vi "Set File Path.vi"(8 "error in":errorcluster) -> (0 "error out":errorcluster, 3 "path":path)   [LabVIEW 2018]
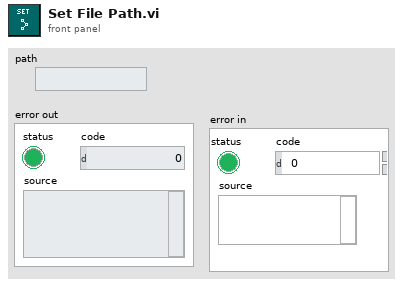
[diagram p1: front panel]
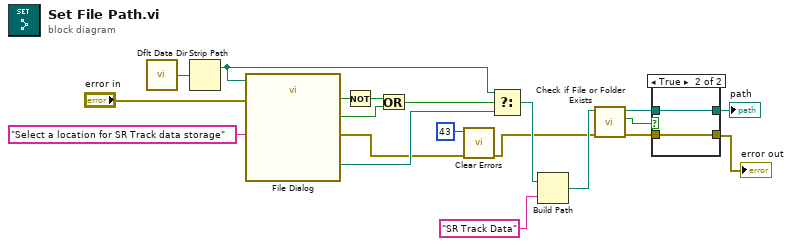
[diagram p0: block diagram]
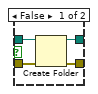
[diagram p2: hidden frame]
diagram:
  n1 = call <vilib>:"Dflt Data Dir.vi"() -> ("App:Default Data Directory"=w10:path)
  n2 = Strip Path(path=w10) -> (stripped path=w5:path)  [unwired: 1 out]
  n3 = call "File Dialog"("start path"=w5, "prompt"="Select a location for SR Track data storage", "error in"="error in") -> ("selected path"=w15:path, "exists"=w9:bool, "cancelled"=w7:bool, "error out"=w4:errorcluster)  [unwired: 9 in]
  n4 = Not(x=w9) -> (.not. x?=w8:bool)
  n5 = Or(x=w8, y=w7) -> (x .or. y?=w6:bool)
  n6 = call <vilib>:"Clear Errors.vi"("error in (no error)"=w4, "specific error code to clear (0: all)"=43) -> ("error out"=w3:errorcluster)  [unwired: 4 in, 1 out]
  n7 = Select(t=w5, s=w6, f=w15) -> (s? t:f=w16:path)
  n8 = Build Path(base path=w16, name or relative path="SR Track Data" ("prompt")) -> (appended path=w17:path)
  n9 = call <vilib>:"Check if File or Folder Exists.vi"("error in (no error)"=w3, "path"=w17) -> ("error out"=w13:errorcluster, "file or folder exists?"=w11:bool, "dup path"=w12:path)  [unwired: 7 in]
  n10 = case shown="True" w11 {
    tunnel: [w24 w25] -> w20
    tunnel: [w23 w26] -> w19
    tunnel: w13 -> [w22 w25]
    tunnel: w12 -> [w21 w26]
    frame False {
      n11 = Create Folder(path (use dialog)=w21, error in=w22) -> (created path=w23:path, error out=w24:errorcluster)  [unwired: 1 in, 1 out]
    }
    frame True {
    }
  }
  "path" <- w19
  "error out" <- w20
